vi "LoggerSetDefault.vi"(8 "error in (no error)":errorcluster, 11 "Connection in":refnum<class "Connection.lvclass">) -> (0 "error out":errorcluster, 3 "Connection out":refnum<class "Connection.lvclass">)   [LabVIEW 2022 SP3, in "Connection.lvlib" / "Connection.lvclass"]
uses:
  Connection.lvclass
  C:/Users/jakub/repos/gh/sw4sys/lv-tcp-server-sample/LoggingActor/Source/LoggingActor/LoggingActor/LoggingActor.lvclass
  Logger/Source/Logger/_Level.ctl
  LoggingActor/Source/LoggingActor/LoggingActor/LoggingActor.lvclass/LoggingActor.ctl
  LoggingActor/Source/LoggingActor/LoggingActor/Write Logger.vi
  Logger/Source/FileHandler/FileHandler.lvclass
  C:/Users/jakub/repos/gh/sw4sys/lv-tcp-server-sample/Logger/Source/Handler/Handler.lvclass
  Logger/Source/Logger/Logger.lvclass
  Connection.lvclass/Connection.ctl
  DateTime/Source/DateTime.lvlib
  Logger/Source/Handler/Handler.lvclass
  C:/Program Files (x86)/National Instruments/LabVIEW 2022/vi.lib/ActorFramework/Actor/Actor.lvclass
  C:/Users/jakub/repos/gh/sw4sys/lv-tcp-server-sample/TcpServerSample/Source/TcpServerSample/Connection/Connection/Connection.lvclass
  C:/Users/jakub/repos/gh/sw4sys/lv-tcp-server-sample/Logger/Source/FileHandler/FileHandler.lvclass
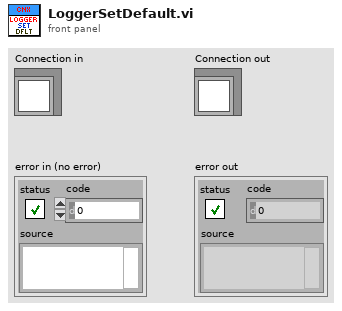
[diagram p1: front panel]
types:
  T1 = typedef "Logger.lvlib/Logger.lvclass/_Level.ctl" = enum16{"NOTSET", "DEBUG", "INFO", "WARNING", "ERROR", "CRITICAL"}
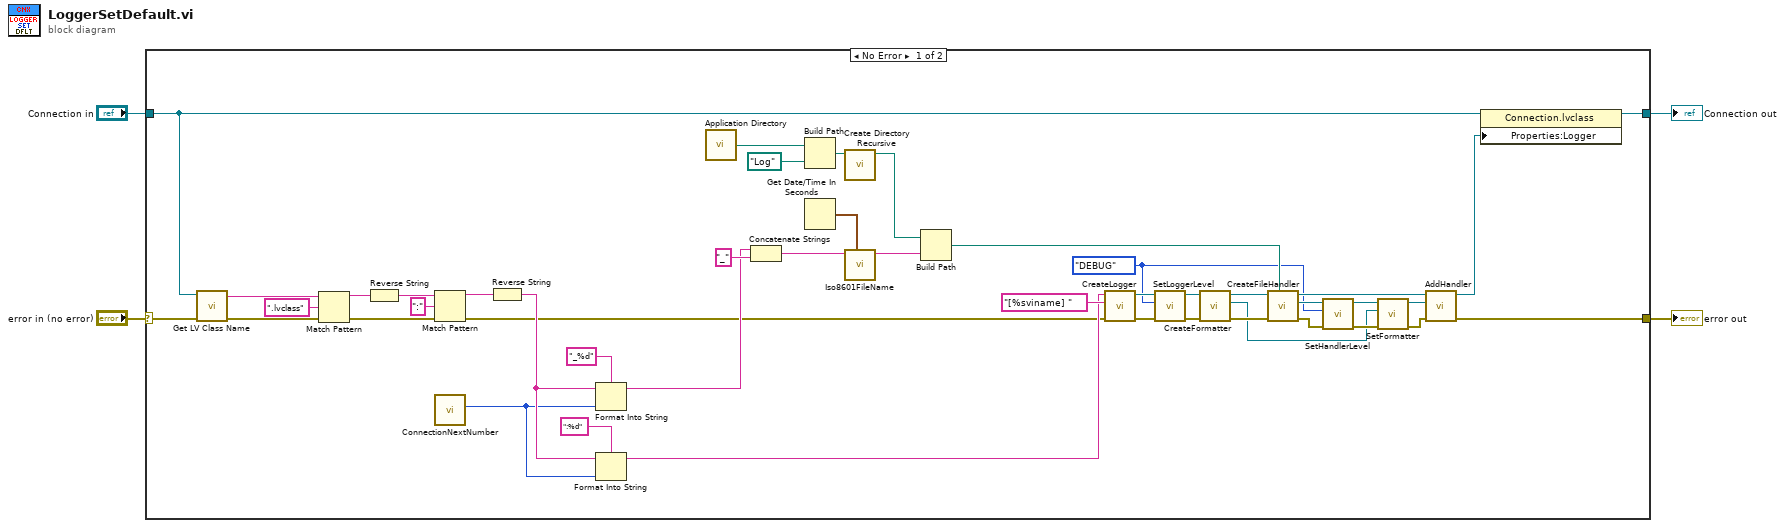
[diagram p0: block diagram]
diagram:
  n1 = case shown="No Error" "error in (no error)" {
    selector: "error in (no error)" -> [w18 w49]
    tunnel: [w17 w49] -> w2
    tunnel: [w12 w48] -> w1
    tunnel: "Connection in" -> [w14 w48]
    frame No Error {
      w25 = _Level."DEBUG" ("Level")
      n2 = call <vilib>:"Get LV Class Name.vi"("error in (no error)"=w18, "object"=w14) -> ("error out"=w5:errorcluster, "class name"=w21:string)  [unwired: 8 in]
      n3 = Match Pattern(string=w21, regular expression=".lvclass") -> (before substring=w23:string)  [unwired: 1 in, 3 out]
      n4 = Reverse String(1:w23) -> (0:w20:string)
      n5 = Match Pattern(string=w20, regular expression=":") -> (before substring=w19:string)  [unwired: 1 in, 3 out]
      n6 = call "ConnectionNextNumber.vi"() -> ("ConnectionNextNumber"=w8:u32)  [unwired: 11 in]
      n7 = Reverse String(1:w19) -> (0:w9:string)
      n8 = Format Into String(format string="_%d", initial string=w9, w8) -> (resulting string=w10:string)  [unwired: 1 in, 1 out]
      n9 = Format Into String(format string=":%d", initial string=w9, w8) -> (resulting string=w6:string)  [unwired: 1 in, 1 out]
      n10 = call <vilib>:"Application Directory.vi"() -> ("Application Directory"=w44:path)
      n11 = Concatenate Strings(w10, "_" ("Prefix ('')")) -> (w37:string)
      n12 = Build Path(base path=w44, name or relative path=path "Log") -> (appended path=w42:path)
      n13 = Get Date/Time In Seconds() -> (seconds since 1Jan1904=w40:timestamp)
      n14 = call <vilib>:"Create Directory Recursive.vi"("directory"=w42) -> ("directory copy"=w39:path)  [unwired: 4 in, 2 out]
      n15 = call "Iso8601FileName.vi"("TimeStamp"=w40, "Prefix ('')"=w37) -> ("FileName"=w41:string)  [unwired: 9 in]
      n16 = Build Path(base path=w39, name or relative path=w41) -> (appended path=w36:path)
      n17 = call "CreateLogger.vi"("error in (no error)"=w5, "MessagePrefixFormat"="[%sviname] ", "Name"=w6) -> ("error out"=w47:errorcluster, "Logger"=w45:refnum<class "Logger.lvclass">)  [unwired: 7 in]
      n18 = call-dynamic "SetLoggerLevel.vi"("error in (no error)"=w47, "Level"=w25, "Logger in"=w45) -> ("error out"=w46:errorcluster, "Logger out"=w30:refnum<class "Logger.lvclass">)  [unwired: 7 in]
      n19 = call-dynamic "CreateFormatter.vi"("error in (no error)"=w46, "Logger in"=w30) -> ("error out"=w31:errorcluster, "Formatter"=w16:refnum<class "Formatter.lvclass">, "Logger out"=w29:refnum<class "Logger.lvclass">)  [unwired: 7 in]
      n20 = call-dynamic "CreateFileHandler.vi"("FIlePath"=w36, "error in (no error)"=w31, "Logger in"=w29) -> ("error out"=w33:errorcluster, "FileHandler"=w35:refnum<class "FileHandler.lvclass">, "Logger out"=w28:refnum<class "Logger.lvclass">)  [unwired: 6 in]
      n21 = call "SetHandlerLevel.vi"("error in (no error)"=w33, "Level"=w25, "Handler in"=w35) -> ("error out"=w32:errorcluster, "Handler out"=w34:refnum<class "Handler.lvclass">)  [unwired: 7 in]
      n22 = call "SetFormatter.vi"("error in (no error)"=w32, "Formatter in"=w16, "Handler in"=w34) -> ("error out"=w26:errorcluster, "Handler out"=w27:refnum<class "Handler.lvclass">)  [unwired: 6 in, 1 out]
      n23 = call-dynamic "AddHandler.vi"("error in (no error)"=w26, "Handler in"=w27, "Logger in"=w28) -> ("error out"=w17:errorcluster, "Logger out"=w13:refnum<class "Logger.lvclass">)  [unwired: 6 in, 1 out]
      n24 = property class="Connection.lvclass"(reference=w14, "Properties:Logger"=w13) -> (reference out=w12:refnum<class "Connection.lvclass">)  [unwired: 1 in, 1 out]
    }
    frame Error {
    }
  }
  "error out" <- w2
  "Connection out" <- w1
